vi "FTW-Messenger-Post.vi"(0 "Messenger":refnum<class "FTW-Messenger.lvclass">, 5 "Message":refnum<class "FTW-Message.lvclass">, 11 "error in":errorcluster) -> (4 "Messenger out":refnum<class "FTW-Messenger.lvclass">, 15 "error out":errorcluster)   [LabVIEW 2014, in "FTW-Messenger.lvclass"]
uses:
  FTW-Messenger.lvclass
  Message/FTW-Message.lvclass
panel:
  # "Inputs"
  # "Outputs"
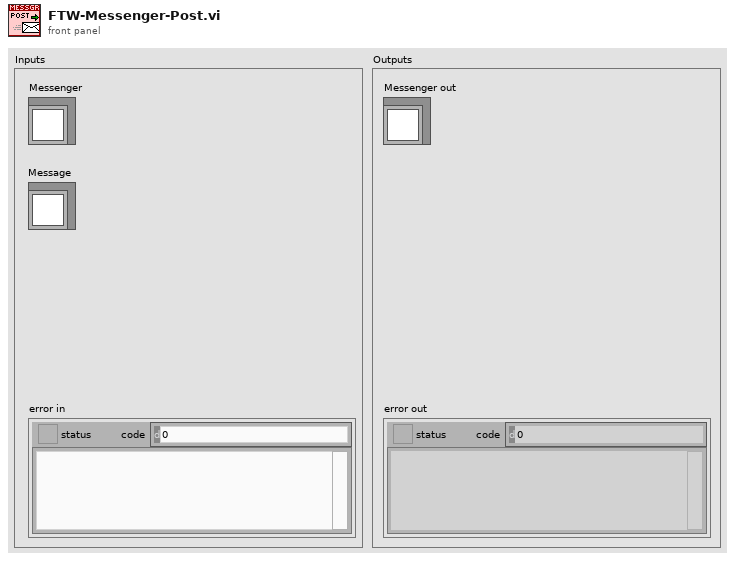
[diagram p1: front panel]
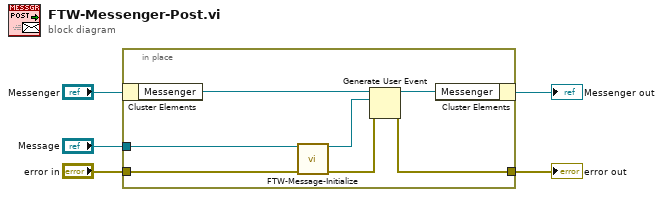
[diagram p0: block diagram]
diagram:
  n1 = in-place {
    in-place-border: [w12] -> w5
    in-place-border: "error in" -> [w7]
    in-place-border: "Message" -> [w9]
    n2 = in-place-cluster #1("Messenger") -> ("Messenger"=w11:refnum<user-event>)
    n3 = call "FTW-Message-Initialize.vi"("Message"=w9, "error in"=w7) -> ("Message out"=w8:refnum<class "FTW-Message.lvclass">, "error out"=w6:errorcluster)  [unwired: 12 in]
    n4 = Generate User Event(user event=w11, event data cluster=w8, error in=w6) -> (user event out=w10:refnum<user-event>, error out=w12:errorcluster)  [unwired: 1 in]
    n5 = in-place-cluster #1("Messenger"=w10) -> (→"Messenger out":refnum<class "FTW-Messenger.lvclass">)
  }
  "error out" <- w5
